vi "Add SmallImages to ListView.vi"(8 "error in (no error)":errorcluster caption="错误输入（无错误）", 10 "ImageFile Path":path[](array[path]), 11 "ListViewClass 输入":refnum<class "ListViewClass.lvclass"> caption="DNL_LabVIEW Object in") -> (0 "error out":errorcluster caption="错误输出", 3 "ListViewClass 输出":refnum<class "ListViewClass.lvclass"> caption="DNL_LabVIEW Object out")   [LabVIEW 2012, in "ListViewClass.lvclass"]
uses:
  ListViewClass.lvclass
  ListViewClass.lvclass/ListViewClass.ctl
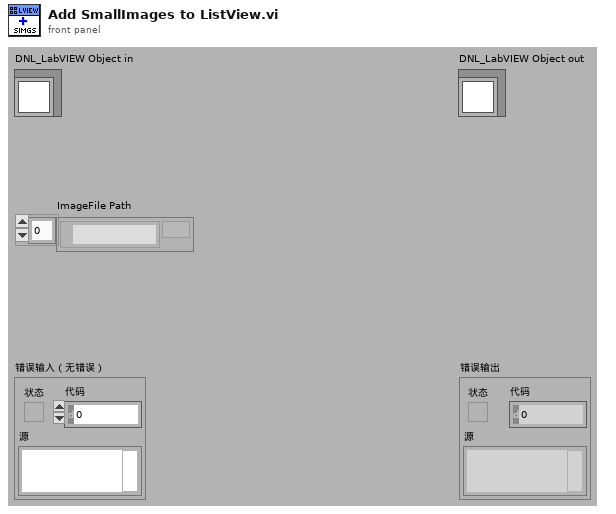
[diagram p1: front panel]
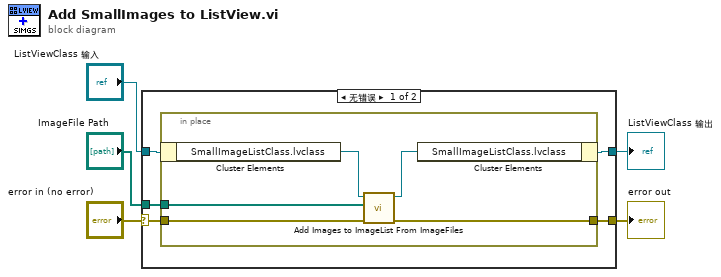
[diagram p0: block diagram]
diagram:
  n1 = case shown="无错误" "error in (no error)" {
    selector: "error in (no error)" -> [w9 w17]
    tunnel: [w8 w17] -> w4
    tunnel: [w6 w16] -> w2
    tunnel: "ListViewClass 输入" -> [w10 w16]
    tunnel: "ImageFile Path" -> [w7 _]
    frame No Error {
      n2 = in-place {
        in-place-border: w9 -> [w13]
        in-place-border: [w12] -> w8
        in-place-border: w7 -> [w11]
        n3 = in-place-cluster #1(w10) -> ("SmallImageListClass.lvclass"=w15:refnum<class "ImageListClass.lvclass">)
        n4 = call "Add Images to ImageList From ImageFiles.vi"("error in (no error)"=w13, "ImageFile Path"=w11, "ImageListClass 输入"=w15) -> ("error out"=w12:errorcluster, "ImageListClass 输出"=w14:refnum<class "ImageListClass.lvclass">)  [unwired: 7 in]
        n5 = in-place-cluster #1("SmallImageListClass.lvclass"=w14) -> (w6:refnum<class "ListViewClass.lvclass">)
      }
    }
    frame Error {
    }
  }
  "error out" <- w4
  "ListViewClass 输出" <- w2
